vi "GVMethodenwechsel_ECD.vi"() -> ()   [LabVIEW 2017]
panel:
  out "Methodenwechsel?":bool
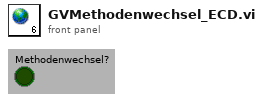
[diagram p1: front panel]
diagram:
